vi "meididor de distancia archivo adicional.vi"(8 "error in":errorcluster) -> (0 "error out":errorcluster, 3 "task out":refnum<k21>)   [LabVIEW 2016]
uses:
  <vilib>/DAQmx/configure/timing.llb/DAQmx Timing (Implicit).vi
  <vilib>/DAQmx/create/channels.llb/DAQmx Create Channel (CO-Pulse Generation-Time).vi
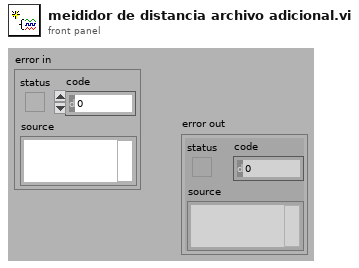
[diagram p1: front panel]
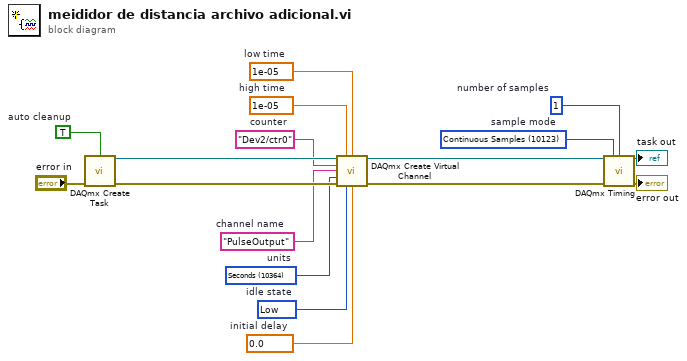
[diagram p0: block diagram]
diagram:
  w1 = 10123 items=["Finite Samples"=10178, "Continuous Samples"=10123, "Hardware Timed Single Point"=12522]  # sample mode
  w2 = 1  # number of samples
  w6 = 1e-05  # low time
  w7 = 1e-05  # high time
  w8 = 0.0  # initial delay
  w9 = 10214 items=["High"=10192, "Low"=10214]  # idle state
  w10 = 10364 items=["Seconds"=10364, "From Custom Scale"=10065]  # units
  w11 = "PulseOutput"  # channel name
  w13 = "Dev2/ctr0"  # counter
  w15 = TRUE  # auto cleanup
  n1 = call <vilib>:"DAQmx Create Task.vi"("auto cleanup"=w15, "error in"="error in") -> ("task out"=w14:refnum<k21>, "error out"=w16:errorcluster)  [unwired: 12 in]
  n2 = call-poly <vilib>:"DAQmx Create Virtual Channel.vi"("task in"=w14, "high time"=w7, "low time"=w6, "counter"=w13, "name to assign"=w11, "units"=w10, "error in"=w16, "idle state"=w9, "initial delay"=w8) -> ("task out"=w3:refnum<k21>, "error out"=w12:errorcluster)  [unwired: 5 in]
  n3 = call-poly <vilib>:"DAQmx Timing.vi"("task/channels in"=w3, "sample mode"=w1, "samples per channel"=w2, "error in"=w12) -> ("task out"=→"task out":refnum<k21>, "error out"=→"error out":errorcluster)  [unwired: 10 in]
